vi "NKT_Config.vi"(8 "entrée d'erreur (pas d'erreur)":errorcluster) -> (0 "sortie d'erreur":errorcluster)   [LabVIEW 2026]
doc: "+--------------------------------------------------------------+\n¦ ÉTAT CONFIG ¦\n¦ ¦\n¦ 1. RegisterWriteU8 — Emission ¦\n¦ PortName : portName (shift register) ¦\n¦ DeviceID : 15 | RegID : 48 | Index : -1 ¦\n¦ Value U8 : cluster ON/OFF ? 3 si TRUE, 0 si FALSE ¦\n¦ ¦\n¦ 2. RegisterWriteU16 — Puissance ¦\n¦ PortName : portName (shift register) ¦\n¦ DeviceID : 15 | RegID : 55 | Index : -1 ¦\n¦ Value U16 : cluster Power × 10 ¦\n¦ ¦\n¦ 3. RegisterWriteU16 — LWP ¦\n¦ PortName : portName (shift register) ¦\n¦ DeviceID : 16 | RegID : 52 | Index : -1 ¦\n¦ Value U16 : Floor(Lambda - Bandwidth/2) × 10 ¦\n¦ ¦\n¦ 4. RegisterWriteU16 — SWP ¦\n¦ PortName : portName (shift register) ¦\n¦ DeviceID : 16 | RegID : 51 | Index : -1 ¦\n¦ Value U16 : Floor(Lambda + Bandwidth/2) × 10 ¦\n¦ ¦\n¦ 5. RegisterWriteU16 — ND ¦\n¦ PortName : portName (shift register) ¦\n¦ DeviceID : 16 | RegID : 32 | Index : -1 ¦\n¦ Value U16 : cluster ND × 10 ¦\n+---------------------------------------------------------------+"
uses:
  Controls/TypeDef_FGV.ctl
  <instrlib>/NKTP_API/NKTP_API.lvlib
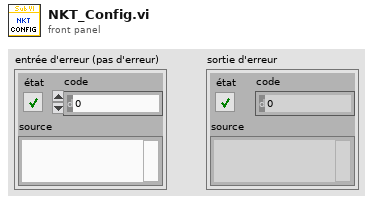
[diagram p1: front panel]
types:
  T1 = typedef "TypeDef_FGV.ctl" = enum16{"Initialize", "Write", "Read"}
  T2 = typedef "Laser.ctl" = cluster{"Emission (ON/OFF)":bool, "Wavelength (nm)":dbl, "Bandwidth (nm)":dbl, "Power (%)":dbl, "ND (%)":dbl}
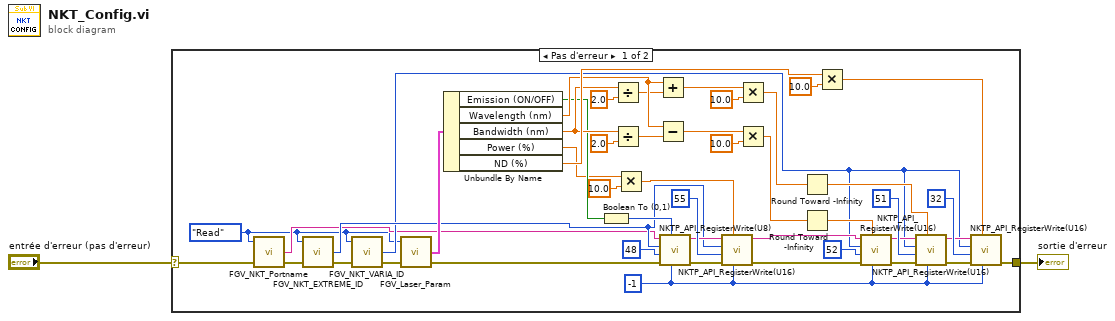
[diagram p0: block diagram]
diagram:
  n1 = case shown="Pas d'erreur" "entrée d'erreur (pas d'erreur)" {
    selector: "entrée d'erreur (pas d'erreur)" -> [w7 w50]
    tunnel: [w47 w50] -> w2
    frame No Error {
      w48 = i16 -1 ("index")
      w4 = TypeDef_FGV."Read" ("Action")
      n2 = call "FGV_NKT_Portname.vi"("error in"=w7, "Action"=w4) -> ("error out"=w6:errorcluster, "Portname"=w5:string)  [unwired: 2 in]
      n3 = call "FGV_NKT_EXTREME_ID.vi"("error in"=w6, "Action"=w4) -> ("error out"=w10:errorcluster, "ID"=w9:i32)  [unwired: 2 in]
      n4 = call "FGV_NKT_VARIA_ID.vi"("error in"=w10, "Action"=w4) -> ("error out"=w11:errorcluster, "ID"=w8:i32)  [unwired: 2 in]
      n5 = call "FGV_Laser_Param.vi"("error in"=w11, "Action"=w4) -> ("error out"=w13:errorcluster, "Laser params"=w12:T2)  [unwired: 2 in]
      n6 = Unbundle By Name(w12) -> ("Emission (ON/OFF)"=w15:bool, "Wavelength (nm)"=w38:dbl, "Bandwidth (nm)"=w39:dbl, "Power (%)"=w3:dbl, "ND (%)"=w44:dbl)
      n7 = Boolean To (0,1)(Boolean=w15) -> (0, 1=w16:i16)
      n8 = Divide(x=w39, y=2.0) -> (x/y=w37:dbl)
      n9 = Divide(x=w39, y=2.0) -> (x/y=w25:dbl)
      n10 = Multiply(x=w3, y=10.0) -> (x*y=w20:dbl)
      n11 = Add(x=w38, y=w37) -> (x+y=w35:dbl)
      n12 = Subtract(x=w38, y=w25) -> (x-y=w27:dbl)
      n13 = call <instrlib>:"NKTP_API_RegisterWrite(U8).vi"("index"=w48, "value"=w16, "error in"=w13, "regId"=u8 48, "devId"=w9, "portname"=w5) -> ("error out"=w18:errorcluster, "portname out"=w17:string)  [unwired: 4 in]
      n14 = call <instrlib>:"NKTP_API_RegisterWrite(U16).vi"("index"=w48, "value"=w20, "error in"=w18, "regId"=u8 55, "devId"=w9, "portname"=w17) -> ("error out"=w23:errorcluster, "portname out"=w22:string)  [unwired: 4 in]
      n15 = Multiply(x=w35, y=10.0) -> (x*y=w33:dbl)
      n16 = Multiply(x=w27, y=10.0) -> (x*y=w29:dbl)
      n17 = Round Toward -Infinity(1:w33) -> (0:w40:dbl)
      n18 = Round Toward -Infinity(1:w29) -> (0:w30:dbl)
      n19 = Multiply(x=w44, y=10.0) -> (x*y=w45:dbl)
      n20 = call <instrlib>:"NKTP_API_RegisterWrite(U16).vi"("index"=w48, "value"=w30, "error in"=w23, "regId"=u8 52, "devId"=w8, "portname"=w22) -> ("error out"=w32:errorcluster, "portname out"=w31:string)  [unwired: 4 in]
      n21 = call <instrlib>:"NKTP_API_RegisterWrite(U16).vi"("index"=w48, "value"=w40, "error in"=w32, "regId"=u8 51, "devId"=w8, "portname"=w31) -> ("error out"=w43:errorcluster, "portname out"=w42:string)  [unwired: 4 in]
      n22 = call <instrlib>:"NKTP_API_RegisterWrite(U16).vi"("index"=w48, "value"=w45, "error in"=w43, "regId"=u8 32, "devId"=w8, "portname"=w42) -> ("error out"=w47:errorcluster)  [unwired: 4 in, 1 out]
    }
    frame Error {
    }
  }
  "sortie d'erreur" <- w2
